vi "Ack Overpressure.vi"(8 "error in (no error)":errorcluster, 11 "ASIA Pump C Settings in":T1) -> (0 "error out":errorcluster)   [LabVIEW 2018, in "ASIA Pump.lvlib"]
uses:
  ASIA Pump.lvlib
  Pump Settings.ctl
panel:
  out "path out":path
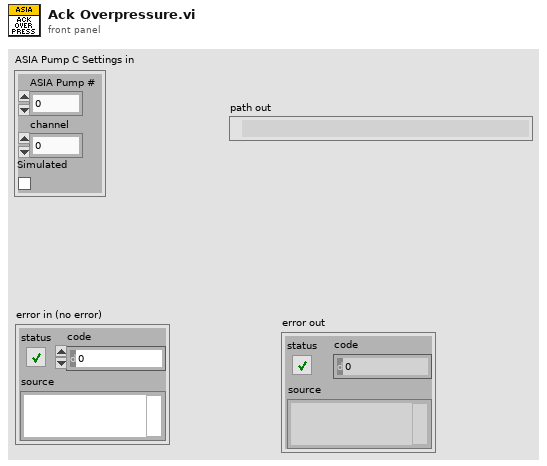
[diagram p1: front panel]
types:
  T1 = typedef "ASIA Pump.lvlib/Pump Settings.ctl" = cluster{"ASIA Pump #":i32, "channel":i32, "Simulated":bool}
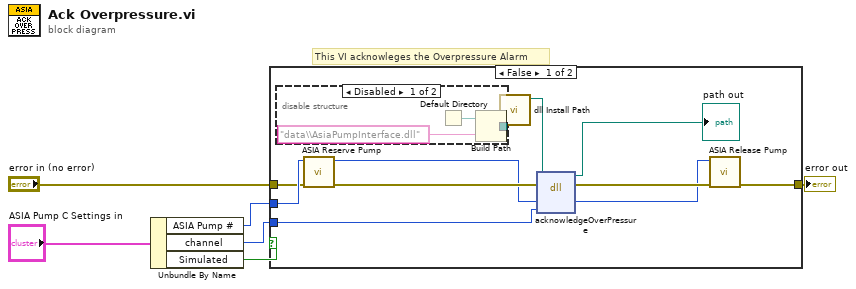
[diagram p0: block diagram]
diagram:
  # "This VI acknowleges the Overpressure Alarm"
  n1 = Unbundle By Name("ASIA Pump C Settings in") -> ("ASIA Pump #"=w4:i32, "channel"=w2:i32, "Simulated"=w5:bool)
  n2 = case shown="False" w5 {
    tunnel: w4 -> [w16 _]
    tunnel: "error in (no error)" -> [w15 w20]
    tunnel: w2 -> [w11 _]
    tunnel: [w9 w20] -> w1
    frame False {
      n3 = disable-structure shown="Disabled" {
        disable-tunnel: [w18 _] -> _
        frame Disabled {
          n4 = Default Directory() -> (w17:path)
          n5 = Build Path(base path=w17, name or relative path="data\\AsiaPumpInterface.dll") -> (appended path=w18:path)
        }
        frame Enabled {
        }
      }
      n6 = call "ASIA Reserve Pump.vi"("error in (no error)"=w15, "ASIA Pump # In"=w16) -> ("error out"=w14:errorcluster, "ASIA Pump # Out"=w10:i32)  [unwired: 8 in]
      n7 = call "dll Install Path.vi"() -> ("system directory"=w8:path)  [unwired: 11 in]
      n8 = dll-call lib="C:/Program Files (x86)/Pfizer/FAST/data/AsiaPumpInterface.dll" fn="acknowledgeOverPressure"(path in=w8, error in=w14, "pumpNum"=w10, "channel"=w11) -> (path out=→"path out":path, error out=w13:errorcluster, "pumpNum"=w12:u32)  [unwired: 3 in]
      n9 = call "ASIA Release Pump.vi"("error in (no error)"=w13, "pumpNum"=w12) -> ("error out"=w9:errorcluster)  [unwired: 8 in, 1 out]
    }
    frame True {
    }
  }
  "error out" <- w1
